vi "GOOP_CheckClassState.vi"(6 "ClassFileMayBeReadOnly(False)":bool, 8 "error in":errorcluster, 11 "Library Refnum":refnum<vi>) -> (0 "error out":errorcluster)   [LabVIEW 2014]
uses:
  <resource>/Framework/Providers/Open_GDS/SubVIs/GOOP_ErrorCodes.ctl
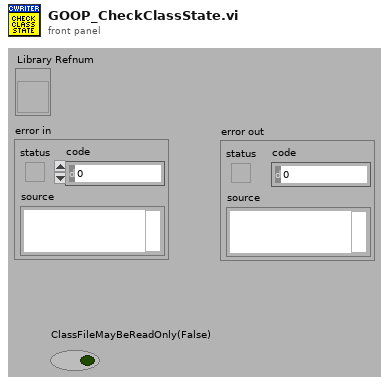
[diagram p1: front panel]
types:
  T1 = typedef "GOOP_ErrorCodes.ctl" = enum16{"LicenseFileMissing", "LicenseFileNotCorrect", "NoProductAccessGranted", "AgreementNoAccepted", "NoValidProviderFound", "LicenseExpired", "LanguageUndefined", "LanguageFileMissing", "LanguageFileChecksumError", "DublicateLanguageTranslation", "LanguageStringIDNotFound", "CommunityLimitReached", "ClassFileLocked", "ClassFileReadOnly", "ProjectNotValid"}
  T2 = enum32{"invalid lock state", "Not Locked", "Locked (No Password)", "Password-protected"}
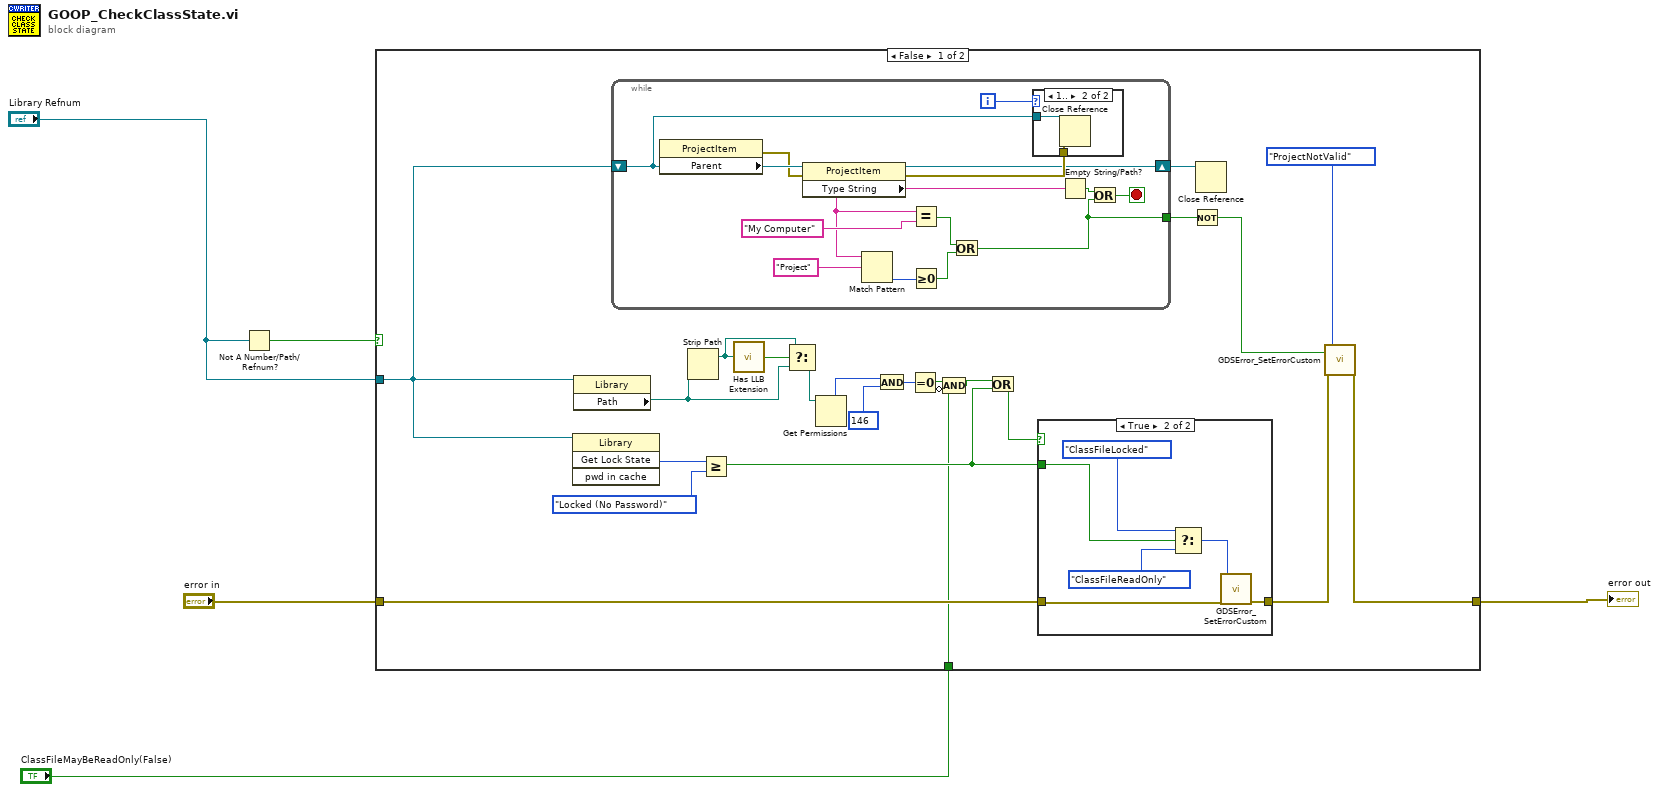
[diagram p0: block diagram]
diagram:
  n1 = Not A Number/Path/Refnum?(number/path/refnum="Library Refnum") -> (NaN/Path/Refnum?=w4:bool)
  n2 = case shown="False" w4 {
    tunnel: "Library Refnum" -> [w6 _]
    tunnel: "error in" -> [w21 w52]
    tunnel: [w13 w52] -> w3
    tunnel: "ClassFileMayBeReadOnly(False)" -> [w10 _]
    frame False {
      n3 = invoke class="Library" method="Get Lock State"(reference=w6) -> ("Get Lock State"=w27:T2)  [unwired: 3 in, 3 out]
      n4 = property class="Library"(reference=w6) -> ("Path"=w17:path)  [unwired: 1 in, 2 out]
      n5 = while {
        shift-right: [w38] -> w8
        shift-left: w6 -> [w35]
        tunnel: [w28] -> w9
        i -> [w34]
        stop <- w37 stop-if-true
        n6 = property class="ProjectItem"(reference=w35) -> (error out=w40:errorcluster, "Parent"=w42:refnum<vi>)  [unwired: 1 in, 1 out]
        n7 = property class="ProjectItem"(reference=w42, error in=w40) -> (reference out=w38:refnum<vi>, error out=w39:errorcluster, "Type String"=w33:string)
        n8 = Match Pattern(string=w33, regular expression="Project") -> (offset past match=w31:i32)  [unwired: 1 in, 3 out]
        n9 = Equal?(x=w33, y="My Computer") -> (x = y?=w29:bool)
        n10 = Greater Or Equal To 0?(x=w31) -> (x >= 0?=w30:bool)
        n11 = Or(x=w29, y=w30) -> (x .or. y?=w28:bool)
        n12 = case shown="1.." w34 {
          tunnel: w39 -> [_ w44]
          tunnel: w35 -> [_ w43]
          frame 0, Default {
          }
          frame 1.. {
            n13 = Close Reference(reference=w43, error in (no error)=w44) -> ()  [unwired: 1 out]
          }
        }
        n14 = Empty String/Path?(string/path=w33) -> (empty?=w41:bool)
        n15 = Or(x=w41, y=w28) -> (x .or. y?=w37:bool)
      }
      n16 = Strip Path(path=w17) -> (stripped path=w18:path)  [unwired: 1 out]
      n17 = Greater Or Equal?(x=w27, y=T2."Locked (No Password)" ("Lock State:Get")) -> (x >= y?=w20:bool)
      n18 = call <vilib>:"Has LLB Extension.vi"("path"=w18) -> ("path to VI library?"=w19:bool)
      n19 = Select(t=w18, s=w19, f=w17) -> (s? t:f=w16:path)
      n20 = Get Permissions(11:w16) -> (5:w25:i16)  [unwired: 1 in, 4 out]
      n21 = And(x=w25, y=i16 146) -> (x .and. y?=w23:i16)
      n22 = Equal To 0?(x=w23) -> (x = 0?=w12:bool)
      n23 = Compound Arithmetic op=AND(w12, invert w10) -> (w11:bool)
      n24 = Or(x=w11, y=w20) -> (x .or. y?=w22:bool)
      n25 = case shown="True" w22 {
        tunnel: w21 -> [w45 w46]
        tunnel: [w45 w51] -> w14
        tunnel: w20 -> [_ w50]
        frame False {
        }
        frame True {
          n26 = Select(t=GOOP_ErrorCodes."ClassFileLocked" ("ErrorCodes"), s=w50, f=GOOP_ErrorCodes."ClassFileReadOnly" ("ErrorCodes")) -> (s? t:f=w47:T1)
          n27 = call <resource>:"GDSError_SetErrorCustom.vi"("error in (no error)"=w46, "UserDefinedCodes(+5000)"=w47) -> ("error out"=w51:errorcluster)  [unwired: 17 in]
        }
      }
      n28 = Not(x=w9) -> (.not. x?=w7:bool)
      n29 = Close Reference(reference=w8) -> ()  [unwired: 1 in, 1 out]
      n30 = call <resource>:"GDSError_SetErrorCustom.vi"("status"=w7, "error in (no error)"=w14, "UserDefinedCodes(+5000)"=GOOP_ErrorCodes."ProjectNotValid" ("ErrorCodes")) -> ("error out"=w13:errorcluster)  [unwired: 16 in]
    }
    frame True {
    }
  }
  "error out" <- w3
